vi "FPGA_DIOReadPWMValue.vi"(8 "error in (no error)":errorcluster, 10 "PWMChannel":T1=enum."PWM 1", 11 "DIODeviceRef In":T2) -> (0 "error out":errorcluster, 2 "PWMValue":u16=127, 3 "DIODeviceRef Out":T2)   [LabVIEW 2017]
uses:
  <vilib>/Rock Robotics/SystemInterfaces/DIO/FPGA_DIODevRef.ctl
  <vilib>/Rock Robotics/SystemInterfaces/DIO/FPGA_DIOPWMChannel.ctl
  <vilib>/Rock Robotics/SystemInterfaces/System/FPGA_SystemFPGA Ref Global.vi
  <vilib>/Utility/error.llb/Error Cluster From Error Code.vi
  <vilib>/rvi/errors/niLvFpgaAdjustHostInterfaceError.vi
  <vilib>/rvi/interface/nirviReadWriteControl/nirviReadWriteControl.xnode
  <vilib>/Rock Robotics/SystemInterfaces/System/FPGA_SystemFRC FPGA Ref.ctl
  <vilib>/rvi/interface/Simulation/niFpgaSimulationCallBeginRW.vi
  NiFpgaLv.dll
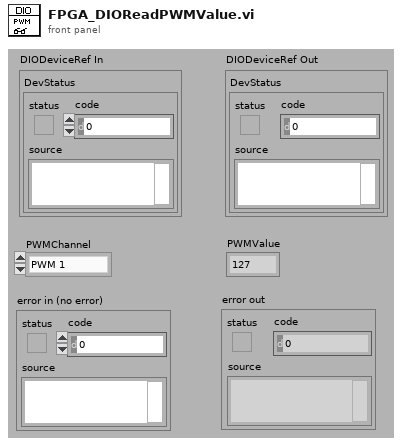
[diagram p1: front panel]
types:
  T1 = typedef "FPGA_DIOPWMChannel.ctl" = enum8{"PWM 0", "PWM 1", "PWM 2", "PWM 3", "PWM 4", "PWM 5", "PWM 6", "PWM 7", "PWM 8", "PWM 9", "PWM MXP 0", "PWM MXP 1", "PWM MXP 2", "PWM MXP 3", "PWM MXP 4", "PWM MXP 5", "PWM MXP 6", "PWM MXP 7", "PWM MXP 8", "PWM MXP 9", "Invalid"}
  T2 = typedef "FPGA_DIODevRef.ctl" = cluster{"DevStatus":errorcluster}
  T3 = typedef "FPGA_SystemFRC FPGA Ref.ctl" = refnum<k20>
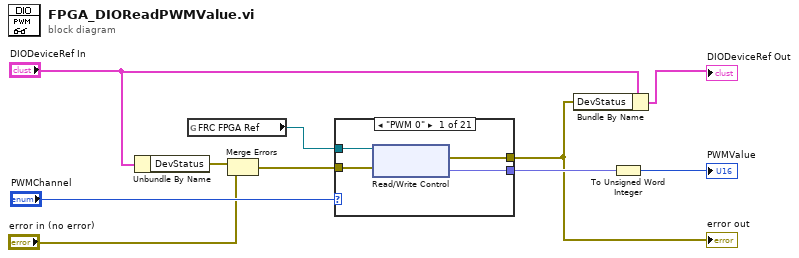
[diagram p0: block diagram]
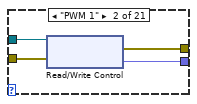
[diagram p2: hidden frame]
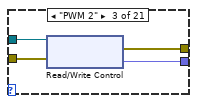
[diagram p3: hidden frame]
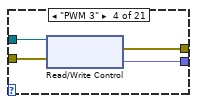
[diagram p4: hidden frame]
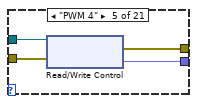
[diagram p5: hidden frame]
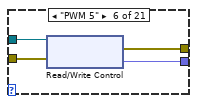
[diagram p6: hidden frame]
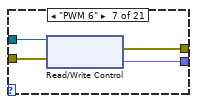
[diagram p7: hidden frame]
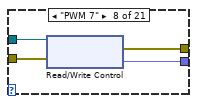
[diagram p8: hidden frame]
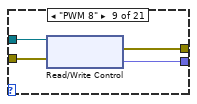
[diagram p9: hidden frame]
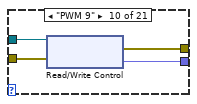
[diagram p10: hidden frame]
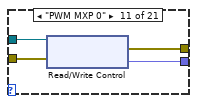
[diagram p11: hidden frame]
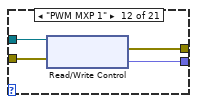
[diagram p12: hidden frame]
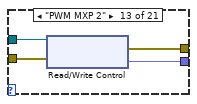
[diagram p13: hidden frame]
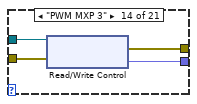
[diagram p14: hidden frame]
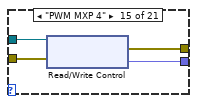
[diagram p15: hidden frame]
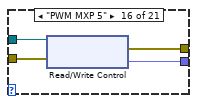
[diagram p16: hidden frame]
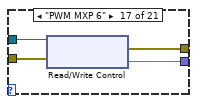
[diagram p17: hidden frame]
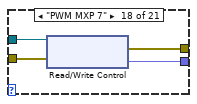
[diagram p18: hidden frame]
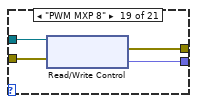
[diagram p19: hidden frame]
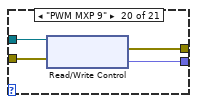
[diagram p20: hidden frame]
diagram:
  n1 = Unbundle By Name("DIODeviceRef In") -> ("DevStatus"=w5:errorcluster)
  n2 = global read "FPGA_SystemFPGA Ref Global.vi" "FRC FPGA Ref"() -> (w1:T3)
  n3 = Merge Errors(w5, "error in (no error)") -> (w4:errorcluster)
  n4 = case shown="\"PWM 0\"" "PWMChannel" {
    tunnel: w1 -> [w12 w16 w20 w24 w28 w32 w36 w40 w44 w48 w52 w56 w60 w64 w68 w72 w76 w80 w84 w88 _]
    tunnel: w4 -> [w13 w17 w21 w25 w29 w33 w37 w41 w45 w49 w53 w57 w61 w65 w69 w73 w77 w81 w85 w89 w92]
    tunnel: [w14 w18 w22 w26 w30 w34 w38 w42 w46 w50 w54 w58 w62 w66 w70 w74 w78 w82 w86 w90 w91] -> w6
    tunnel: [w11 w15 w19 w23 w27 w31 w35 w39 w43 w47 w51 w55 w59 w63 w67 w71 w75 w79 w83 w87 _] -> w9
    frame "PWM 0" {
      n5 = xnode "Read/Write Control"("FPGA VI Reference In"=w12, "error in"=w13) -> ("error out"=w14:errorcluster, "PWM.Hdr0"=w11:fxp<+,12,12>)  [unwired: 1 out]
    }
    frame "PWM 1" {
      n6 = xnode "Read/Write Control"("FPGA VI Reference In"=w16, "error in"=w17) -> ("error out"=w18:errorcluster, "PWM.Hdr1"=w15:fxp<+,12,12>)  [unwired: 1 out]
    }
    frame "PWM 2" {
      n7 = xnode "Read/Write Control"("FPGA VI Reference In"=w20, "error in"=w21) -> ("error out"=w22:errorcluster, "PWM.Hdr2"=w19:fxp<+,12,12>)  [unwired: 1 out]
    }
    frame "PWM 3" {
      n8 = xnode "Read/Write Control"("FPGA VI Reference In"=w24, "error in"=w25) -> ("error out"=w26:errorcluster, "PWM.Hdr3"=w23:fxp<+,12,12>)  [unwired: 1 out]
    }
    frame "PWM 4" {
      n9 = xnode "Read/Write Control"("FPGA VI Reference In"=w28, "error in"=w29) -> ("error out"=w30:errorcluster, "PWM.Hdr4"=w27:fxp<+,12,12>)  [unwired: 1 out]
    }
    frame "PWM 5" {
      n10 = xnode "Read/Write Control"("FPGA VI Reference In"=w32, "error in"=w33) -> ("error out"=w34:errorcluster, "PWM.Hdr5"=w31:fxp<+,12,12>)  [unwired: 1 out]
    }
    frame "PWM 6" {
      n11 = xnode "Read/Write Control"("FPGA VI Reference In"=w36, "error in"=w37) -> ("error out"=w38:errorcluster, "PWM.Hdr6"=w35:fxp<+,12,12>)  [unwired: 1 out]
    }
    frame "PWM 7" {
      n12 = xnode "Read/Write Control"("FPGA VI Reference In"=w40, "error in"=w41) -> ("error out"=w42:errorcluster, "PWM.Hdr7"=w39:fxp<+,12,12>)  [unwired: 1 out]
    }
    frame "PWM 8" {
      n13 = xnode "Read/Write Control"("FPGA VI Reference In"=w44, "error in"=w45) -> ("error out"=w46:errorcluster, "PWM.Hdr8"=w43:fxp<+,12,12>)  [unwired: 1 out]
    }
    frame "PWM 9" {
      n14 = xnode "Read/Write Control"("FPGA VI Reference In"=w48, "error in"=w49) -> ("error out"=w50:errorcluster, "PWM.Hdr9"=w47:fxp<+,12,12>)  [unwired: 1 out]
    }
    frame "PWM MXP 0" {
      n15 = xnode "Read/Write Control"("FPGA VI Reference In"=w52, "error in"=w53) -> ("error out"=w54:errorcluster, "PWM.MXP0"=w51:fxp<+,12,12>)  [unwired: 1 out]
    }
    frame "PWM MXP 1" {
      n16 = xnode "Read/Write Control"("FPGA VI Reference In"=w56, "error in"=w57) -> ("error out"=w58:errorcluster, "PWM.MXP1"=w55:fxp<+,12,12>)  [unwired: 1 out]
    }
    frame "PWM MXP 2" {
      n17 = xnode "Read/Write Control"("FPGA VI Reference In"=w60, "error in"=w61) -> ("error out"=w62:errorcluster, "PWM.MXP2"=w59:fxp<+,12,12>)  [unwired: 1 out]
    }
    frame "PWM MXP 3" {
      n18 = xnode "Read/Write Control"("FPGA VI Reference In"=w64, "error in"=w65) -> ("error out"=w66:errorcluster, "PWM.MXP3"=w63:fxp<+,12,12>)  [unwired: 1 out]
    }
    frame "PWM MXP 4" {
      n19 = xnode "Read/Write Control"("FPGA VI Reference In"=w68, "error in"=w69) -> ("error out"=w70:errorcluster, "PWM.MXP4"=w67:fxp<+,12,12>)  [unwired: 1 out]
    }
    frame "PWM MXP 5" {
      n20 = xnode "Read/Write Control"("FPGA VI Reference In"=w72, "error in"=w73) -> ("error out"=w74:errorcluster, "PWM.MXP5"=w71:fxp<+,12,12>)  [unwired: 1 out]
    }
    frame "PWM MXP 6" {
      n21 = xnode "Read/Write Control"("FPGA VI Reference In"=w76, "error in"=w77) -> ("error out"=w78:errorcluster, "PWM.MXP6"=w75:fxp<+,12,12>)  [unwired: 1 out]
    }
    frame "PWM MXP 7" {
      n22 = xnode "Read/Write Control"("FPGA VI Reference In"=w80, "error in"=w81) -> ("error out"=w82:errorcluster, "PWM.MXP7"=w79:fxp<+,12,12>)  [unwired: 1 out]
    }
    frame "PWM MXP 8" {
      n23 = xnode "Read/Write Control"("FPGA VI Reference In"=w84, "error in"=w85) -> ("error out"=w86:errorcluster, "PWM.MXP8"=w83:fxp<+,12,12>)  [unwired: 1 out]
    }
    frame "PWM MXP 9" {
      n24 = xnode "Read/Write Control"("FPGA VI Reference In"=w88, "error in"=w89) -> ("error out"=w90:errorcluster, "PWM.MXP9"=w87:fxp<+,12,12>)  [unwired: 1 out]
    }
    frame "Invalid" {
      n25 = call <vilib>:"FPGA_DIOERRInvalidPWMChannel.vi"("error in (no error)"=w92) -> ("error out"=w91:errorcluster)
    }
  }
  "error out" <- w6
  n26 = Bundle By Name(cluster="DIODeviceRef In", "DevStatus"=w6) -> (→"DIODeviceRef Out":T2)
  n27 = To Unsigned Word Integer(number=w9) -> (unsigned 16bit integer=→"PWMValue":u16)
